vi "题目5.vi"() -> ()   [LabVIEW 2017]
panel:
  out "日期/时间字符串":string
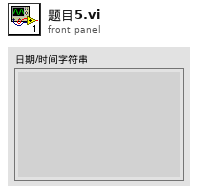
[diagram p1: front panel]
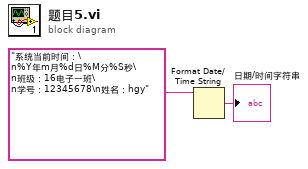
[diagram p0: block diagram]
diagram:
  n1 = Format Date/Time String(time format string (%c)="系统当前时间：\n%Y年m月%d日%M分%S秒\n班级：16电子一班\n学号：12345678\n姓名：hgy" ("时间格式字符串(%c)")) -> (date/time string=→"日期/时间字符串":string)  [unwired: 2 in]
